vi "add_elementToHostMessages.vi"(0 "Host_Reference":refnum<class "HGF_Reference.lvclass">, 2 "timeout in ms (-1)":i32=-1, 3 "MoAgSy_Message":refnum<class "MoAgSy_Message.lvclass">, 5 "error in (no error)":errorcluster) -> (14 "dup Host_Reference":refnum<class "HGF_Reference.lvclass">, 19 "error out":errorcluster)   [LabVIEW 2009, in "MoAgSy.lvlib" / "MoAgSy_Host.lvclass"]
doc: "<B>public</B> VI enqueues new host messages to referenced hosts internal queue.\n\nF.Berck@gsi.de\nGSI Darmstadt 2009"
uses:
  MoAgSy_Host.lvclass
  HGF_BaseClasses/HGF_Reference/HGF_Reference.lvclass
  MoAgSy_Message/MoAgSy_Message.lvclass
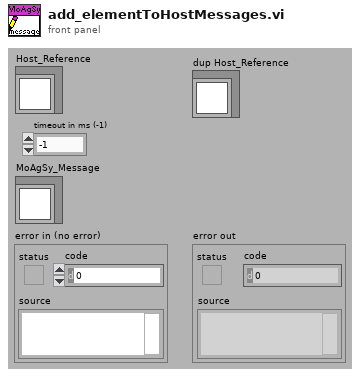
[diagram p1: front panel]
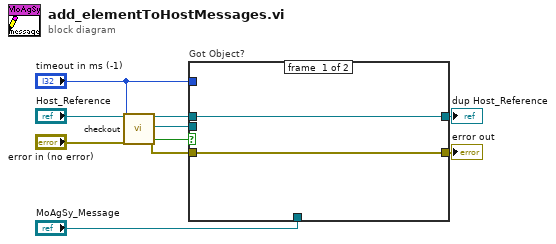
[diagram p0: block diagram]
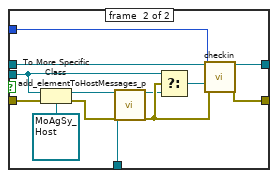
[diagram p2: hidden frame]
diagram:
  n1 = call "checkout.vi"("HGF_Reference"="Host_Reference", "timeout in ms (-1)"="timeout in ms (-1)", "error in (no error)"="error in (no error)") -> ("dup HGF_Reference"=w7:refnum<class "HGF_Reference.lvclass">, "Object"=w9:refnum<class>, "got object?"=w8:bool, "error out"=w10:errorcluster)  [unwired: 13 out]
  n2 = case "Got Object?" shown="True" w8 {
    tunnel: w9 -> [_ w13]
    tunnel: w7 -> [w12 w23]
    tunnel: [w12 w22] -> w3
    tunnel: "timeout in ms (-1)" -> [_ w21]
    tunnel: [w11 w20] -> w4
    tunnel: w10 -> [w11 w19]
    tunnel: "MoAgSy_Message" -> [_ w16]
    frame #0 {
    }
    frame #1 {
      n3 = To More Specific Class(target class=refnum<class "MoAgSy_Host.lvclass"> refnum ("MoAgSy.lvlib:MoAgSy_Host.lvclass"), reference=w13, error in=w19) -> (specific class reference=w18:refnum<class "MoAgSy_Host.lvclass">, error out=w17:errorcluster)
      n4 = call "add_elementToHostMessages_p.vi"("MoAgSy_Host"=w18, "MoAgSy_Message"=w16, "error in (no error)"=w17) -> ("dup MoAgSy_Host"=w15:refnum<class "MoAgSy_Host.lvclass">, "error out"=w25:errorcluster)  [unwired: 15 out]
      n5 = Select(t=w13, s=w25, f=w15) -> (s? t:f=w14:refnum<class>)
      n6 = call "checkin.vi"("HGF_Reference"=w23, "Object"=w14, "timeout /ms (-1)"=w21, "error in (no error)"=w25) -> ("dup HGF_Reference"=w22:refnum<class "HGF_Reference.lvclass">, "error out"=w20:errorcluster)  [unwired: 14 out]
    }
  }
  "dup Host_Reference" <- w3
  "error out" <- w4
